vi "oa_Buffered Output Resampled Data (N Channels).vi"(0 "resampled signal in":cluster{"r0":dbl, "dr":dbl, "Y":dbl[]}[](array[cluster]) {"r0" format="%.2p"; "dr" format="%.2p"; "Y" format="%.2f"}, 1 "reset? (True)":bool=TRUE, 7 "interpolated pulse positions":dbl[](array[numeric]) format="%.2f", 9 "display revolutions":cluster{"start [rev]":dbl, "duration [rev]":dbl}={"start [rev]"=0.0, "duration [rev]"=1.0} {"duration [rev]" format="%.2f"; "start [rev]" format="%.2f"}, 11 "error in":errorcluster) -> (4 "resampled signal out":cluster{"r0":dbl, "dr":dbl, "Y":dbl[]}[](array[cluster]) {"r0" format="%.2p"; "dr" format="%.2p"; "Y" format="%.2f"}, 8 "interpolated pulse positions out":dbl[](array[numeric]), 15 "error out":errorcluster)   [LabVIEW 2017]
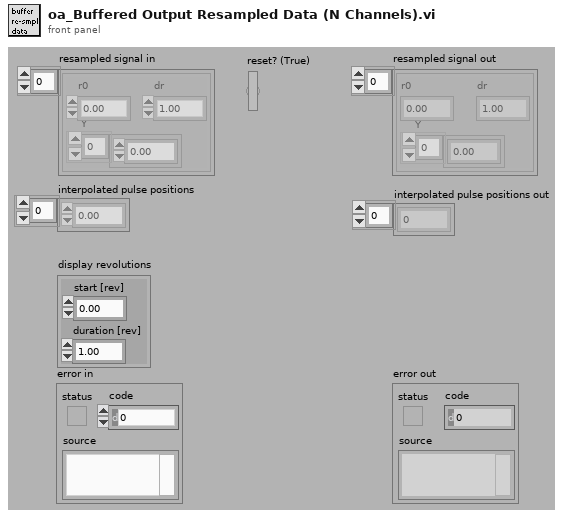
[diagram p1: front panel]
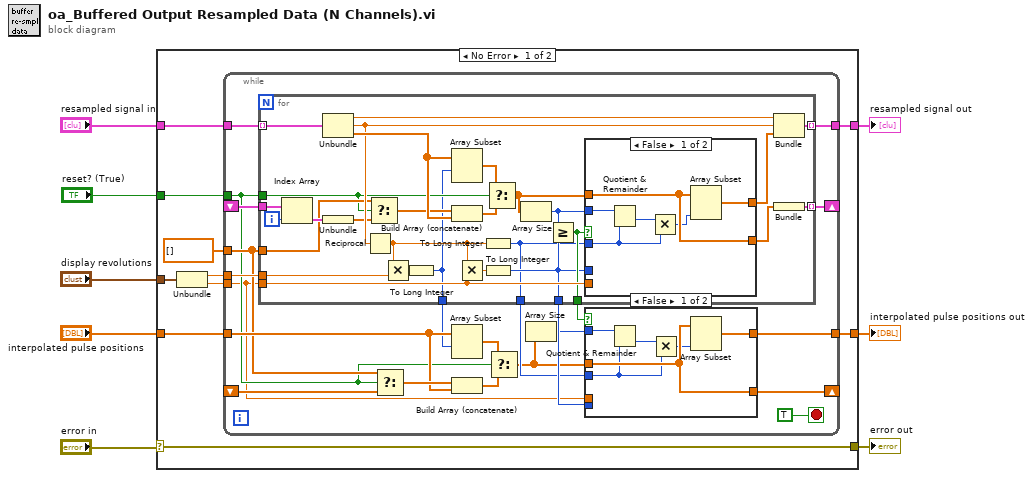
[diagram p0: block diagram]
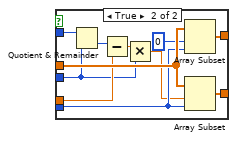
[diagram p2: hidden frame]
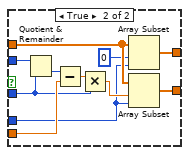
[diagram p3: hidden frame]
diagram:
  n1 = case shown="No Error" "error in" {
    selector: "error in" -> [w18 w105]
    tunnel: [w18 w105] -> w7
    tunnel: "resampled signal in" -> [w17 w104]
    tunnel: "display revolutions" -> [w16 _]
    tunnel: "reset? (True)" -> [w15 _]
    tunnel: [w12 w104] -> w3
    tunnel: "interpolated pulse positions" -> [w10 w103]
    tunnel: [w9 w103] -> w1
    frame No Error {
      n2 = Unbundle(w16) -> ("start [rev]"=w14:dbl, "duration [rev]"=w13:dbl)
      n3 = while {
        tunnel: w17 -> [w39]
        tunnel: w15 -> [w28]
        tunnel: w14 -> [w38]
        tunnel: w13 -> [w19]
        tunnel: [w37] -> w12
        shift-right: [w36] -> _
        shift-left: _ -> [w35]
        tunnel: dbl[] [] ("t") -> [w30]
        tunnel: w10 -> [w31]
        shift-right: [w25] -> _
        shift-left: _ -> [w27]
        tunnel: [w24] -> w9
        stop <- TRUE stop-if-true
        n4 = for {
          tunnel: w39 -> [w85] mode=indexing
          tunnel: w28 -> [w62]
          tunnel: w38 -> [w84]
          tunnel: w19 -> [w72]
          tunnel: [w74] -> w37 mode=indexing
          tunnel: [w69] -> w36 mode=indexing
          tunnel: w35 -> [w68]
          tunnel: w30 -> [w63]
          tunnel: [w61] -> w29
          tunnel: [w60] -> w26
          tunnel: [w59] -> w23
          tunnel: [w58] -> w22
          i -> [w67]
          n5 = Index Array(array=w68, index=w67) -> (element=w66:cluster{dbl[]})
          n6 = Unbundle(w85) -> ("r0"=w75:dbl, "dr"=w76:dbl, "Y"=w81:dbl[])
          n7 = Unbundle(w66) -> (w65:dbl[])
          n8 = Reciprocal(x=w76) -> (1/x=w73:dbl)
          n9 = Select(t=w63, s=w62, f=w65) -> (s? t:f=w64:dbl[])
          n10 = Multiply(x=w73, y=w84) -> (x*y=w83:dbl)
          n11 = To Long Integer(number=w83) -> (32bit integer=w61:i32)
          n12 = Array Subset(array=w81, index=w61) -> (w82:dbl[])  [unwired: 1 in]
          n13 = Build Array (concatenate)(w64, w81) -> (w80:dbl[])
          n14 = Multiply(x=w73, y=w72) -> (x*y=w71:dbl)
          n15 = To Long Integer(number=w73) -> (32bit integer=w58:i32)
          n16 = To Long Integer(number=w71) -> (32bit integer=w59:i32)
          n17 = Select(t=w82, s=w62, f=w80) -> (s? t:f=w79:dbl[])
          n18 = Array Size(array=w79) -> (size(s)=w78:i32)
          n19 = Greater Or Equal?(x=w78, y=w59) -> (x >= y?=w60:bool)
          n20 = case shown="False" w60 {
            tunnel: w79 -> [w88 w98]
            tunnel: [w88 w97] -> w70
            tunnel: w78 -> [w91 w102]
            tunnel: w58 -> [w89 w95]
            tunnel: [w87 w99] -> w77
            tunnel: w72 -> [_ w100]
            tunnel: w59 -> [_ w92]
            frame False {
              n21 = Quotient & Remainder(x=w91, y=w89) -> (floor(x/y)=w90:i32)  [unwired: 1 out]
              n22 = Multiply(x=w90, y=w89) -> (x*y=w86:i32)
              n23 = Array Subset(array=w88, length=w86) -> (w87:dbl[])  [unwired: 1 in]
            }
            frame True {
              n24 = Quotient & Remainder(x=w102, y=w95) -> (floor(x/y)=w101:i32)  [unwired: 1 out]
              n25 = Subtract(x=w101, y=w100) -> (x-y=w96:dbl)
              n26 = Multiply(x=w96, y=w95) -> (x*y=w93:dbl)
              n27 = Array Subset(array=w98, index=0, length=w92) -> (w99:dbl[])
              n28 = Array Subset(array=w98, index=w93, length=w92) -> (w97:dbl[])
            }
          }
          n29 = Bundle("r0"=w75, "dr"=w76, w77) -> (w74:cluster{"r0":dbl, "dr":dbl, dbl[]})  [unwired: 1 in]
          n30 = Bundle(w70) -> (w69:cluster{dbl[]})  [unwired: 1 in]
        }
        n31 = Select(t=w30, s=w28, f=w27) -> (s? t:f=w34:dbl[])
        n32 = Array Subset(array=w31, index=w29) -> (w32:dbl[])  [unwired: 1 in]
        n33 = Build Array (concatenate)(w34, w31) -> (w33:dbl[])
        n34 = Select(t=w32, s=w28, f=w33) -> (s? t:f=w21:dbl[])
        n35 = Array Size(array=w21) -> (size(s)=w20:i32)
        n36 = case shown="False" w26 {
          tunnel: w21 -> [w46 w56]
          tunnel: [w46 w55] -> w25
          tunnel: [w45 w57] -> w24
          tunnel: w23 -> [_ w54]
          tunnel: w22 -> [w42 w49]
          tunnel: w20 -> [w44 w52]
          tunnel: w19 -> [_ w50]
          frame False {
            n37 = Quotient & Remainder(x=w44, y=w42) -> (floor(x/y)=w43:i32)  [unwired: 1 out]
            n38 = Multiply(x=w43, y=w42) -> (x*y=w41:i32)
            n39 = Array Subset(array=w46, length=w41) -> (w45:dbl[])  [unwired: 1 in]
          }
          frame True {
            n40 = Quotient & Remainder(x=w52, y=w49) -> (floor(x/y)=w51:i32)  [unwired: 1 out]
            n41 = Subtract(x=w51, y=w50) -> (x-y=w48:dbl)
            n42 = Multiply(x=w48, y=w49) -> (x*y=w47:dbl)
            n43 = Array Subset(array=w56, index=0, length=w54) -> (w57:dbl[])
            n44 = Array Subset(array=w56, index=w47, length=w54) -> (w55:dbl[])
          }
        }
      }
    }
    frame Error {
    }
  }
  "error out" <- w7
  "resampled signal out" <- w3
  "interpolated pulse positions out" <- w1
